vi "ATSh_QueryCapability.vi"(4 "Hex_Input":u32 format="%.0x", 6 "Used HexInput (TestMode)":bool, 9 "Value":u32, 10 "ATS_Query":T1, 11 "HandleIn":u32) -> (0 "Return Code":u32, 1 "ReturnValue":u32, 2 "Hex_Request":u32 format="%.0x", 3 "HandleOut":u32)   [LabVIEW 2010]
doc: "_____AlazarTech, Scope_____\n\nQuery information from hardware."
uses:
  ATS_ctl/ATS_Query.ctl
  ATSApi.dll
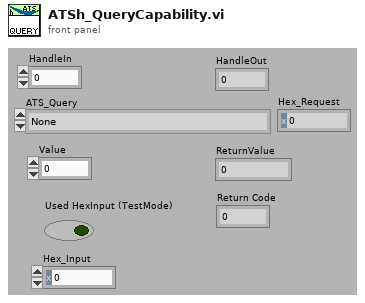
[diagram p1: front panel]
types:
  T1 = typedef "ATS_Query.ctl" = enum16{"None", "NUMBER_OF_RECORDS", "PRETRIGGER_AMOUNT", "RECORD_LENGTH", "TRIGGER_ENGINE", "TRIGGER_DELAY", "TRIGGER_TIMEOUT", "SAMPLE_RATE", "CONFIGURATION_MODE", "DATA_WIDTH", "AUTO_CALIBRATE", "TRIGGER_XXXXX", "CLOCK_SOURCE", "CLOCK_SLOPE", "IMPEDANCE", "INPUT_RANGE", "COUPLING", "MAX_TIMEOUTS_ALLOWED", "ATS_OPERATING_MODE", "CLOCK_DECIMATION_EXTERNAL", "LED_CONTROL", "ATTENUATOR_RELAY", "EXT_TRIGGER_COUPLING", "EXT_TRIGGER_ATTENUATOR_RELAY", "TRIGGER_ENGINE_SOURCE", "TRIGGER_ENGINE_SLOPE", "SEND_DAC_VALUE", "SLEEP_DEVICE", "MEMORY_SIZE", "BOARD_TYPE", "ASOPC_TYPE", "SERIAL_NUMBER", "FIRSTCAL_DATE", "LATEST_CAL_DATE", "LATEST_TEST_DATE"}
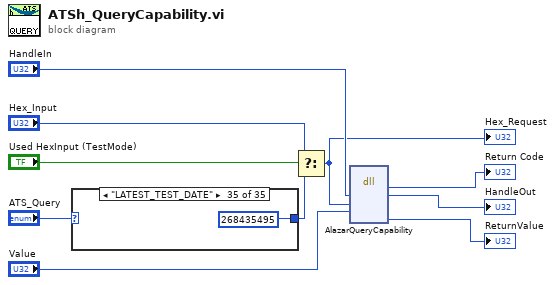
[diagram p0: block diagram]
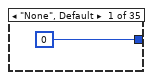
[diagram p2: hidden frame]
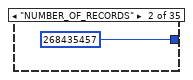
[diagram p3: hidden frame]
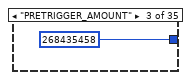
[diagram p4: hidden frame]
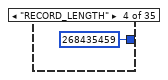
[diagram p5: hidden frame]
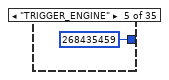
[diagram p6: hidden frame]
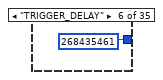
[diagram p7: hidden frame]
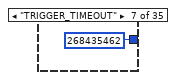
[diagram p8: hidden frame]
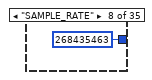
[diagram p9: hidden frame]
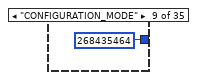
[diagram p10: hidden frame]
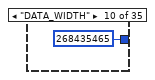
[diagram p11: hidden frame]
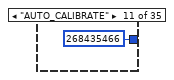
[diagram p12: hidden frame]
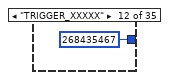
[diagram p13: hidden frame]
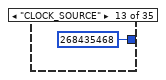
[diagram p14: hidden frame]
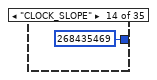
[diagram p15: hidden frame]
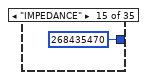
[diagram p16: hidden frame]
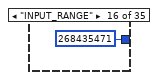
[diagram p17: hidden frame]
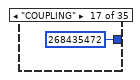
[diagram p18: hidden frame]
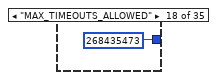
[diagram p19: hidden frame]
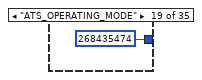
[diagram p20: hidden frame]
diagram:
  n1 = case shown="\"LATEST_TEST_DATE\"" "ATS_Query" {
    tunnel: [u32 0 u32 268435457 u32 268435458 u32 268435459 u32 268435459 u32 268435461 u32 268435462 u32 268435463 u32 268435464 u32 268435465 u32 268435466 u32 268435467 u32 268435468 u32 268435469 u32 268435470 u32 268435471 u32 268435472 u32 268435473 u32 268435474 u32 268435475 u32 268435476 u32 268435480 u32 268435482 u32 268435484 u32 268435486 u32 268435488 u32 268435489 u32 268435490 u32 268435498 u32 268435499 u32 268435500 u32 268435492 u32 268435493 u32 268435494 u32 268435495] -> w5
    frame "None", Default {
    }
    frame "NUMBER_OF_RECORDS" {
    }
    frame "PRETRIGGER_AMOUNT" {
    }
    frame "RECORD_LENGTH" {
    }
    frame "TRIGGER_ENGINE" {
    }
    frame "TRIGGER_DELAY" {
    }
    frame "TRIGGER_TIMEOUT" {
    }
    frame "SAMPLE_RATE" {
    }
    frame "CONFIGURATION_MODE" {
    }
    frame "DATA_WIDTH" {
    }
    frame "AUTO_CALIBRATE" {
    }
    frame "TRIGGER_XXXXX" {
    }
    frame "CLOCK_SOURCE" {
    }
    frame "CLOCK_SLOPE" {
    }
    frame "IMPEDANCE" {
    }
    frame "INPUT_RANGE" {
    }
    frame "COUPLING" {
    }
    frame "MAX_TIMEOUTS_ALLOWED" {
    }
    frame "ATS_OPERATING_MODE" {
    }
    frame "CLOCK_DECIMATION_EXTERNAL" {
    }
    frame "LED_CONTROL" {
    }
    frame "ATTENUATOR_RELAY" {
    }
    frame "EXT_TRIGGER_COUPLING" {
    }
    frame "EXT_TRIGGER_ATTENUATOR_RELAY" {
    }
    frame "TRIGGER_ENGINE_SOURCE" {
    }
    frame "TRIGGER_ENGINE_SLOPE" {
    }
    frame "SEND_DAC_VALUE" {
    }
    frame "SLEEP_DEVICE" {
    }
    frame "MEMORY_SIZE" {
    }
    frame "BOARD_TYPE" {
    }
    frame "ASOPC_TYPE" {
    }
    frame "SERIAL_NUMBER" {
    }
    frame "FIRSTCAL_DATE" {
    }
    frame "LATEST_CAL_DATE" {
    }
    frame "LATEST_TEST_DATE" {
    }
  }
  n2 = Select(t="Hex_Input", s="Used HexInput (TestMode)", f=w5) -> (s? t:f=w3:u32)
  "Hex_Request" <- w3
  n3 = dll-call lib="ATSApi.dll" fn="AlazarQueryCapability"("h"="HandleIn", "Request"=w3, "Value"="Value") -> (→"Return Code":u32, "h"=→"HandleOut":u32, "ReturnValue"=→"ReturnValue":u32)  [unwired: 6 in, 2 out]
